vi "UPDATE LIST VIEW.vi"(10 "COLUMNS TO VIEW":bool, 11 "REFERENCES":T1) -> ()   [LabVIEW 2019]
uses:
  Controls/References Cluster.ctl
  <vilib>/userDefined/High Color/IMAQdx.ctl
  Controls/Custom Calendar/Custom Calendar.xctl
  Controls/Column Names/Inventory Column Names.ctl
  Controls/Column Names/User Column Names.ctl
  Controls/Column Names/Inventory Archive Column Names.ctl
  Controls/Column Names/User Archive Column Names.ctl
  Controls/Column Names/Checked In Archive Column Names.ctl
  Controls/Column Names/Sales Tracking Column Names.ctl
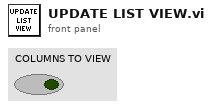
[diagram p1: front panel]
types:
  T1 = typedef "References Cluster.ctl" = cluster{"MAIN PAGES":refnum<vi>, "ADD/EDIT ITEM REFERENCES":cluster{"Identifier":refnum<vi>, "BYU ICN #":refnum<vi>, "Item Description":refnum<vi>, "Comments":refnum<vi>, "Checked Out Date":refnum<vi>, "Due Date":refnum<vi>, "Check Out Location":refnum<vi>, "Reminder Count":refnum<vi>, "Most Recent Reminder Date":refnum<vi>, "BYU ID #":refnum<vi>, "Building/Room":refnum<vi>, "Location in Room":refnum<vi>, "Manual":refnum<vi>, "Manufacturer":refnum<vi>, "Model #":refnum<vi>, "Serial #":refnum<vi>, "Date Acquired":refnum<vi>, "ADD/EDIT ITEM LABEL":refnum<vi>, "ARCHIVE ITEM":refnum<vi>, "Archive Item Inputs":refnum<vi>, "Reminder Notes":refnum<vi>}, "ADD/EDIT USER REFERENCES":cluster{"BYU ID # (##-###-####)":refnum<vi>, "First Name":refnum<vi>, "Last Name":refnum<vi>, "Phone Number (###-###-####)":refnum<vi>, "Email":refnum<vi>, "Department":refnum<vi>, "Graduation Status":refnum<vi>, "Anticipated Graduation Year":refnum<vi>, "Credit Score":refnum<vi>, "Date Added":refnum<vi>, "Graduation Clearance Date":refnum<vi>, "Picture File Name":refnum<vi>, "ADD/EDIT USER LABEL":refnum<vi>, "Department Map":refnum<vi>, "Status Map":refnum<vi>, "Anticipated Graduation Year Map":refnum<vi>, "User Agreement":refnum<vi>, "User Comments":refnum<vi>, "Camera":refnum<vi>}, "RETURN ITEM REFERENCES":cluster{"Item or Person:":refnum<vi>, "Search Return Results":refnum<vi>, "What are you searching for?":refnum<vi>}, "SEARCH DATABASE REFERENCES":cluster{"What to Search For:":refnum<vi>, "Where to Search":refnum<vi>, "Column to Search In":refnum<vi>, "Column to Sort By":refnum<vi>, "Search Database Results":refnum<vi>, "Inventory Column Selector":refnum<vi>, "User Column Selector":refnum<vi>, "Inventory Archive Column Selector":refnum<vi>, "User Archive Column Selector":refnum<vi>, "Sales Tracking Column Selector":refnum<vi>, "Checked In Archive Column Selector":refnum<vi>, "Restore User":refnum<vi>, "Date Range":refnum<vi>, "Dates Less Than":refnum<vi>, "Dates Greater Than":refnum<vi>, "Search Print Receipt":refnum<vi>, "Edit Sale Description":refnum<vi>}, "USER ITEMS REFERENCES":cluster{"USER'S INFORMATION":refnum<vi>, "User's Checked Out Items":refnum<vi>, "User Info Comments":refnum<vi>, "SEE USER INFO COMMENTS":refnum<vi>}, "EDIT ITEMS REFERENCES":cluster{"New Check Out Location":refnum<vi>, "Items to Edit":refnum<vi>, "Edit Items Due Date":refnum<vi>, "New Reminder Notes":refnum<vi>, "New Item Description":refnum<vi>}, "CHECK OUT ITEMS REFERENCES":cluster{"Enter Item:":refnum<vi>, "Check Out Items Due Date":refnum<vi>, "Check Out Location":refnum<vi>, "Items to be Checked Out":refnum<vi>, "Possible Items":refnum<vi>}, "TRANSFER ITEMS REFERENCES":cluster{"Search Parameter":refnum<vi>, "What to Match":refnum<vi>, "Matching Individuals":refnum<vi>, "Items to be Transferred":refnum<vi>}, "SETTINGS REFERENCES":cluster{"PSC Database Settings":refnum<vi>, "PSC Sales Item Spreadsheet":refnum<vi>}, "PSC SALES REFERENCES":cluster{"BYU ID CARD #":refnum<vi>, "Sale Description":refnum<vi>, "Scan or Enter Item Name":refnum<vi>, "Items to be Sold":refnum<vi>, "Grand Total":refnum<vi>, "Item List":refnum<vi>}}
  T2 = cluster{"What to Search For:":refnum<vi>, "Where to Search":refnum<vi>, "Column to Search In":refnum<vi>, "Column to Sort By":refnum<vi>, "Search Database Results":refnum<vi>, "Inventory Column Selector":refnum<vi>, "User Column Selector":refnum<vi>, "Inventory Archive Column Selector":refnum<vi>, "User Archive Column Selector":refnum<vi>, "Sales Tracking Column Selector":refnum<vi>, "Checked In Archive Column Selector":refnum<vi>, "Restore User":refnum<vi>, "Date Range":refnum<vi>, "Dates Less Than":refnum<vi>, "Dates Greater Than":refnum<vi>, "Search Print Receipt":refnum<vi>, "Edit Sale Description":refnum<vi>}
  T3 = typedef "Inventory Column Names.ctl" = string[]
  T4 = typedef "User Column Names.ctl" = string[]
  T5 = typedef "Inventory Archive Column Names.ctl" = string[]
  T6 = typedef "User Archive Column Names.ctl" = string[]
  T7 = typedef "Checked In Archive Column Names.ctl" = string[]
  T8 = typedef "Sales Tracking Column Names.ctl" = string[]
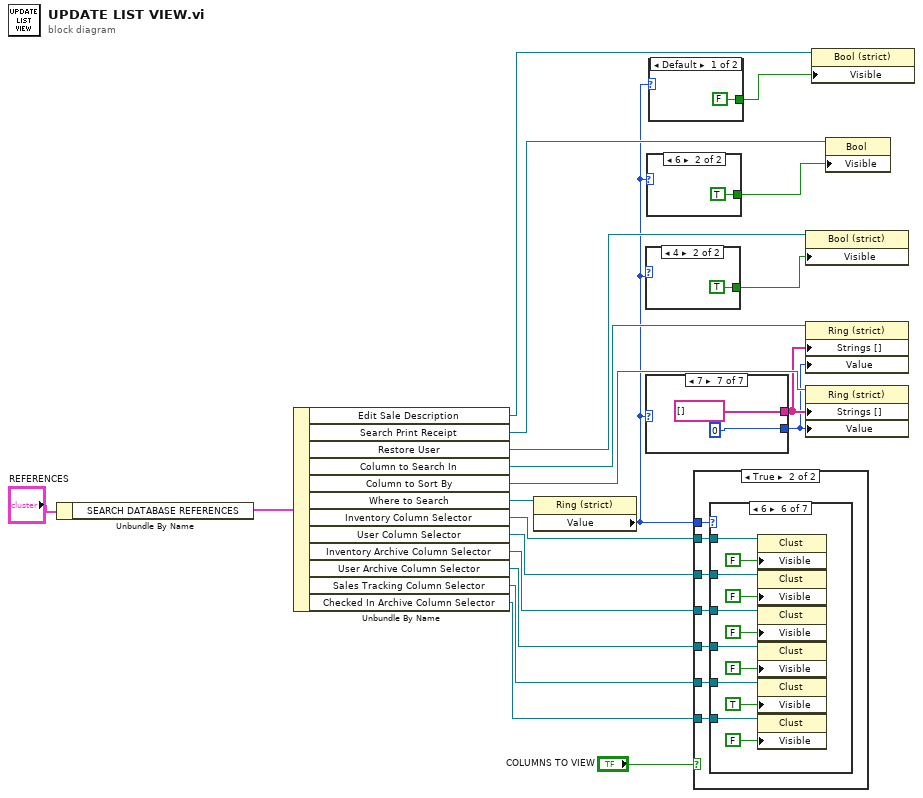
[diagram p0: block diagram]
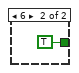
[diagram p2: hidden frame]
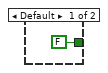
[diagram p3: hidden frame]
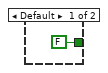
[diagram p4: hidden frame]
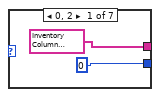
[diagram p5: hidden frame]
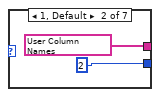
[diagram p6: hidden frame]
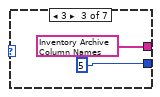
[diagram p7: hidden frame]
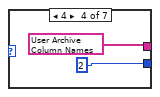
[diagram p8: hidden frame]
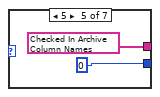
[diagram p9: hidden frame]
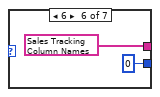
[diagram p10: hidden frame]
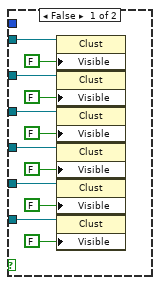
[diagram p11: hidden frame]
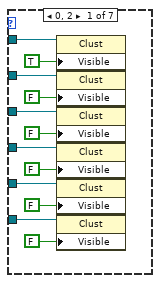
[diagram p12: hidden frame]
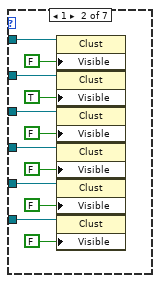
[diagram p13: hidden frame]
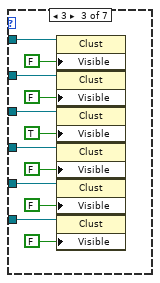
[diagram p14: hidden frame]
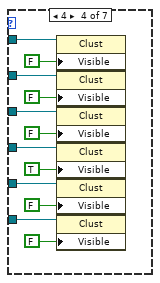
[diagram p15: hidden frame]
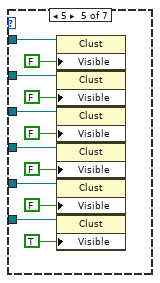
[diagram p16: hidden frame]
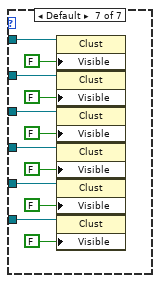
[diagram p17: hidden frame]
diagram:
  n1 = Unbundle By Name("REFERENCES") -> ("SEARCH DATABASE REFERENCES"=w20:T2)
  n2 = Unbundle By Name(w20) -> ("Edit Sale Description"=w3:refnum<vi>, "Search Print Receipt"=w4:refnum<vi>, "Restore User"=w7:refnum<vi>, "Column to Search In"=w11:refnum<vi>, "Column to Sort By"=w10:refnum<vi>, "Where to Search"=w19:refnum<vi>, "Inventory Column Selector"=w18:refnum<vi>, "User Column Selector"=w17:refnum<vi>, "Inventory Archive Column Selector"=w16:refnum<vi>, "User Archive Column Selector"=w15:refnum<vi>, "Sales Tracking Column Selector"=w14:refnum<vi>, "Checked In Archive Column Selector"=w13:refnum<vi>)
  n3 = property class="Ring (strict)"(reference=w19) -> ("Value"=w1:u16)  [unwired: 1 in, 2 out]
  n4 = case shown="4" w1 {
    tunnel: [FALSE ("Visible") TRUE ("Visible")] -> w6
    frame Default {
    }
    frame 4 {
    }
  }
  n5 = case shown="7" w1 {
    tunnel: [T3 ["ME #/ID #", "BYU ICN #", "Item Description", "Comments", "Checked Out Date", "Due Date", "Check Out Location", "Reminder Count", "Most Recent Reminder Date", "BYU ID #", "Building/Room", "Location in Room", "Manual", "Manufacturer", "Model #", "Serial #", "Date Acquired", "Reminder Notes", "First Name", "Last Name"] ("INVENTORY COLUMN NAMES") T4 ["BYU ID #", "First Name", "Last Name", "Phone Number", "Email", "Department", "Graduation Status", "Anticipated Graduation Year", "Credit Score", "Date Added", "Graduation Clearance Date", "User Profile Picture Path"] ("USER COLUMN NAMES") T5 ["Date Disposed", "Disposal Method", "Auction #", "Date Inventory Office Emailed", "Disposal Notes", "Identifier", "BYU ICN #", "Item Description", "Comments", "Building/Room", "Location in Room", "Manual", "Manufacturer", "Model #", "Serial #", "Date Acquired"] ("INVENTORY ARCHIVE COLUMN NAMES") T6 ["BYU ID #", "First Name", "Last Name", "Phone Number", "Email", "Department", "Graduation Status", "Anticipated Graduation Year", "Credit Score", "Date Added", "Graduation Clearance Date", "User Picture File Name", "Date Archived"] ("USER ARCHIVE COLUMN NAMES") T7 ["Identifier", "BYU ICN #", "Item Description", "Comments", "Checked Out Date", "Due Date", "Check Out Location", "Reminder Count", "Most Recent Reminder Date", "BYU ID #", "Building/Room", "Location in Room", "Manual", "Manufacturer", "Model #", "Serial #", "Date Acquired", "Date Returned", "Reminder Notes", "First Name", "Last Name"] ("CHECKED IN ARCHIVE COLUMN NAMES") T8 ["SALE ID #", "BYU ID CARD #", "Sale Description", "Grand Total", "Sale Date", "Item Description", "Item Quantity", "Item Unit Price", "Item Total Price", "Sale Semester"] ("Sales Tracking Column Names") string[] []] -> w9
    tunnel: [u16 0 u16 2 u16 5 u16 2 u16 0 u16 0 u16 0] -> w8
    frame 0, 2 {
    }
    frame 1, Default {
    }
    frame 3 {
    }
    frame 4 {
    }
    frame 5 {
    }
    frame 6 {
    }
    frame 7 {
    }
  }
  n6 = case shown="6" w1 {
    tunnel: [FALSE ("Visible") TRUE ("Visible")] -> w5
    frame Default {
    }
    frame 6 {
    }
  }
  n7 = case shown="Default" w1 {
    tunnel: [FALSE ("Visible") TRUE ("Visible")] -> w2
    frame Default {
    }
    frame 6 {
    }
  }
  n8 = case shown="True" "COLUMNS TO VIEW" {
    tunnel: w1 -> [_ w60]
    tunnel: w18 -> [w47 w59]
    tunnel: w17 -> [w46 w58]
    tunnel: w16 -> [w45 w57]
    tunnel: w15 -> [w44 w56]
    tunnel: w14 -> [w43 w55]
    tunnel: w13 -> [w42 w54]
    frame False {
      n9 = property class="Clust"(reference=w47, "Visible"=FALSE) -> ()  [unwired: 1 in, 2 out]
      n10 = property class="Clust"(reference=w46, "Visible"=FALSE) -> ()  [unwired: 1 in, 2 out]
      n11 = property class="Clust"(reference=w45, "Visible"=FALSE) -> ()  [unwired: 1 in, 2 out]
      n12 = property class="Clust"(reference=w44, "Visible"=FALSE) -> ()  [unwired: 1 in, 2 out]
      n13 = property class="Clust"(reference=w43, "Visible"=FALSE) -> ()  [unwired: 1 in, 2 out]
      n14 = property class="Clust"(reference=w42, "Visible"=FALSE) -> ()  [unwired: 1 in, 2 out]
    }
    frame True {
      n15 = case shown="6" w60 {
        tunnel: w59 -> [w72 w84 w96 w108 w120 w132 w144]
        tunnel: w58 -> [w71 w83 w95 w107 w119 w131 w143]
        tunnel: w57 -> [w70 w82 w94 w106 w118 w130 w142]
        tunnel: w56 -> [w69 w81 w93 w105 w117 w129 w141]
        tunnel: w55 -> [w68 w80 w92 w104 w116 w128 w140]
        tunnel: w54 -> [w67 w79 w91 w103 w115 w127 w139]
        frame 0, 2 {
          n16 = property class="Clust"(reference=w72, "Visible"=TRUE) -> ()  [unwired: 1 in, 2 out]
          n17 = property class="Clust"(reference=w71, "Visible"=FALSE) -> ()  [unwired: 1 in, 2 out]
          n18 = property class="Clust"(reference=w70, "Visible"=FALSE) -> ()  [unwired: 1 in, 2 out]
          n19 = property class="Clust"(reference=w69, "Visible"=FALSE) -> ()  [unwired: 1 in, 2 out]
          n20 = property class="Clust"(reference=w68, "Visible"=FALSE) -> ()  [unwired: 1 in, 2 out]
          n21 = property class="Clust"(reference=w67, "Visible"=FALSE) -> ()  [unwired: 1 in, 2 out]
        }
        frame 1 {
          n22 = property class="Clust"(reference=w84, "Visible"=FALSE) -> ()  [unwired: 1 in, 2 out]
          n23 = property class="Clust"(reference=w83, "Visible"=TRUE) -> ()  [unwired: 1 in, 2 out]
          n24 = property class="Clust"(reference=w82, "Visible"=FALSE) -> ()  [unwired: 1 in, 2 out]
          n25 = property class="Clust"(reference=w81, "Visible"=FALSE) -> ()  [unwired: 1 in, 2 out]
          n26 = property class="Clust"(reference=w80, "Visible"=FALSE) -> ()  [unwired: 1 in, 2 out]
          n27 = property class="Clust"(reference=w79, "Visible"=FALSE) -> ()  [unwired: 1 in, 2 out]
        }
        frame 3 {
          n28 = property class="Clust"(reference=w96, "Visible"=FALSE) -> ()  [unwired: 1 in, 2 out]
          n29 = property class="Clust"(reference=w95, "Visible"=FALSE) -> ()  [unwired: 1 in, 2 out]
          n30 = property class="Clust"(reference=w94, "Visible"=TRUE) -> ()  [unwired: 1 in, 2 out]
          n31 = property class="Clust"(reference=w93, "Visible"=FALSE) -> ()  [unwired: 1 in, 2 out]
          n32 = property class="Clust"(reference=w92, "Visible"=FALSE) -> ()  [unwired: 1 in, 2 out]
          n33 = property class="Clust"(reference=w91, "Visible"=FALSE) -> ()  [unwired: 1 in, 2 out]
        }
        frame 4 {
          n34 = property class="Clust"(reference=w108, "Visible"=FALSE) -> ()  [unwired: 1 in, 2 out]
          n35 = property class="Clust"(reference=w107, "Visible"=FALSE) -> ()  [unwired: 1 in, 2 out]
          n36 = property class="Clust"(reference=w106, "Visible"=FALSE) -> ()  [unwired: 1 in, 2 out]
          n37 = property class="Clust"(reference=w105, "Visible"=TRUE) -> ()  [unwired: 1 in, 2 out]
          n38 = property class="Clust"(reference=w104, "Visible"=FALSE) -> ()  [unwired: 1 in, 2 out]
          n39 = property class="Clust"(reference=w103, "Visible"=FALSE) -> ()  [unwired: 1 in, 2 out]
        }
        frame 5 {
          n40 = property class="Clust"(reference=w120, "Visible"=FALSE) -> ()  [unwired: 1 in, 2 out]
          n41 = property class="Clust"(reference=w119, "Visible"=FALSE) -> ()  [unwired: 1 in, 2 out]
          n42 = property class="Clust"(reference=w118, "Visible"=FALSE) -> ()  [unwired: 1 in, 2 out]
          n43 = property class="Clust"(reference=w117, "Visible"=FALSE) -> ()  [unwired: 1 in, 2 out]
          n44 = property class="Clust"(reference=w116, "Visible"=FALSE) -> ()  [unwired: 1 in, 2 out]
          n45 = property class="Clust"(reference=w115, "Visible"=TRUE) -> ()  [unwired: 1 in, 2 out]
        }
        frame 6 {
          n46 = property class="Clust"(reference=w132, "Visible"=FALSE) -> ()  [unwired: 1 in, 2 out]
          n47 = property class="Clust"(reference=w131, "Visible"=FALSE) -> ()  [unwired: 1 in, 2 out]
          n48 = property class="Clust"(reference=w130, "Visible"=FALSE) -> ()  [unwired: 1 in, 2 out]
          n49 = property class="Clust"(reference=w129, "Visible"=FALSE) -> ()  [unwired: 1 in, 2 out]
          n50 = property class="Clust"(reference=w128, "Visible"=TRUE) -> ()  [unwired: 1 in, 2 out]
          n51 = property class="Clust"(reference=w127, "Visible"=FALSE) -> ()  [unwired: 1 in, 2 out]
        }
        frame Default {
          n52 = property class="Clust"(reference=w144, "Visible"=FALSE) -> ()  [unwired: 1 in, 2 out]
          n53 = property class="Clust"(reference=w143, "Visible"=FALSE) -> ()  [unwired: 1 in, 2 out]
          n54 = property class="Clust"(reference=w142, "Visible"=FALSE) -> ()  [unwired: 1 in, 2 out]
          n55 = property class="Clust"(reference=w141, "Visible"=FALSE) -> ()  [unwired: 1 in, 2 out]
          n56 = property class="Clust"(reference=w140, "Visible"=FALSE) -> ()  [unwired: 1 in, 2 out]
          n57 = property class="Clust"(reference=w139, "Visible"=FALSE) -> ()  [unwired: 1 in, 2 out]
        }
      }
    }
  }
  n58 = property class="Bool (strict)"(reference=w7, "Visible"=w6) -> ()  [unwired: 1 in, 2 out]
  n59 = property class="Ring (strict)"(reference=w11, "Strings []"=w9, "Value"=w8) -> ()  [unwired: 1 in, 2 out]
  n60 = property class="Ring (strict)"(reference=w10, "Strings []"=w9, "Value"=w8) -> ()  [unwired: 1 in, 2 out]
  n61 = property class="Bool (strict)"(reference=w3, "Visible"=w2) -> ()  [unwired: 1 in, 2 out]
  n62 = property class="Bool"(reference=w4, "Visible"=w5) -> ()  [unwired: 1 in, 2 out]
